vi "Open Image.vi"(8 "error in (no error)":errorcluster, 11 "Image":path) -> (0 "error out":errorcluster, 3 "image data":T1)   [LabVIEW 2014, in "Image Comparison.lvclass"]
uses:
  Image Comparison.lvclass
  <vilib>/Utility/error.llb/Error Cluster From Error Code.vi
  <vilib>/ErrorRing/Error Ring.xnode
  <vilib>/picture/picture.llb/imagedata.ctl
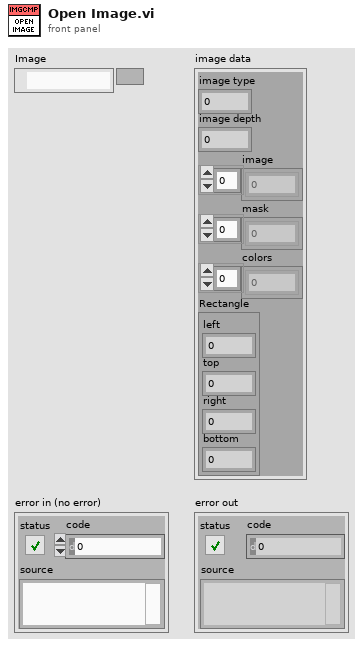
[diagram p1: front panel]
types:
  T1 = typedef "imagedata.ctl" = cluster{"image type":i32, "image depth":i32, "image":u8[], "mask":u8[], "colors":u32[], "Rectangle":cluster{"left":i16, "top":i16, "right":i16, "bottom":i16}}
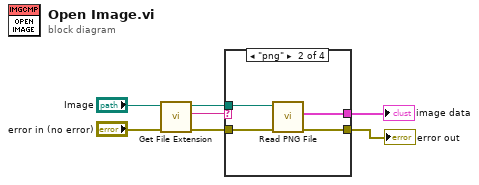
[diagram p0: block diagram]
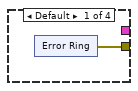
[diagram p2: hidden frame]
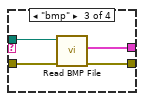
[diagram p3: hidden frame]
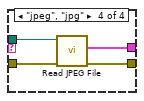
[diagram p4: hidden frame]
diagram:
  n1 = call <vilib>:"Get File Extension.vi"("error in (no error)"="error in (no error)", "file"="Image") -> ("error out"=w6:errorcluster, "lowercase file extension"=w4:string, "dup file"=w5:path)  [unwired: 5 in, 2 out]
  n2 = case shown="\"png\"" w4 {
    tunnel: w5 -> [_ w17 w21 w25]
    tunnel: w6 -> [_ w16 w20 w24]
    tunnel: [_ w15 w19 w23] -> w7
    tunnel: [w8 w14 w18 w22] -> w1
    frame Default {
      n3 = xnode "Error Ring"() -> ("error out"=w8:errorcluster)
    }
    frame "png" {
      n4 = call <vilib>:"Read PNG File.vi"("error in (no error)"=w16, "path to PNG file"=w17) -> ("error out"=w14:errorcluster, "image data"=w15:T1)  [unwired: 7 in, 1 out]
    }
    frame "bmp" {
      n5 = call <vilib>:"Read BMP File.vi"("error in (no error)"=w20, "path to BMP file"=w21) -> ("error out"=w18:errorcluster, "image data"=w19:T1)  [unwired: 7 in, 1 out]
    }
    frame "jpeg", "jpg" {
      n6 = call <vilib>:"Read JPEG File.vi"("error in (no error)"=w24, "path to JPEG file"=w25) -> ("error out"=w22:errorcluster, "image data"=w23:T1)  [unwired: 7 in, 1 out]
    }
  }
  "image data" <- w7
  "error out" <- w1
